vi "2D_scan.vi"(0 "X起始":dbl format="%#_13g", 1 "ERR X":errorcluster, 2 "模块路径":path=path "D:/Github/Motor_ctrl/3d_plot.py", 3 "ERR Y":errorcluster, 4 "Y起始":dbl format="%#_13g", 5 "X步长":dbl format="%#_13g", 6 "Y步长":dbl format="%#_13g", 9 "X终止":dbl format="%#_13g", 10 "Y终止":dbl format="%#_13g", 11 "COM X":refnum<visa-resource-name>, 12 "COM Keithley":refnum<visa-resource-name>, 14 "ERR Keithley":errorcluster, 15 "COM Y":refnum<visa-resource-name>) -> (13 "3D Plot lvclass Array out":refnum<class "3D Plot Datatype.lvclass">[](array[class]) caption="三维曲线lv类数组输出")   [LabVIEW 2018]
uses:
  <vilib>/Math Plots/3D Math Plots/3D Contour/3D Contour XCtrl/3D Contour.xctl
  <vilib>/Math Plots/3D Math Plots/3D Plot/3D Plot Datatype/3D Plot Datatype.lvclass
  <vilib>/Math Plots/3D Math Plots/3D Contour/3D Contour Datatype/Public/Plot Helper (Vector).vi
  <instrlib>/Keithley 648X Series/Keithley 648X Series.lvlib
  <vilib>/Math Plots/3D Math Plots/3D Contour/3D Contour Datatype/3D Contour Datatype.lvclass
panel:
  out "3D Contour":refnum<class "3D Plot Datatype.lvclass">[](xcontrol) caption="三维等高线"
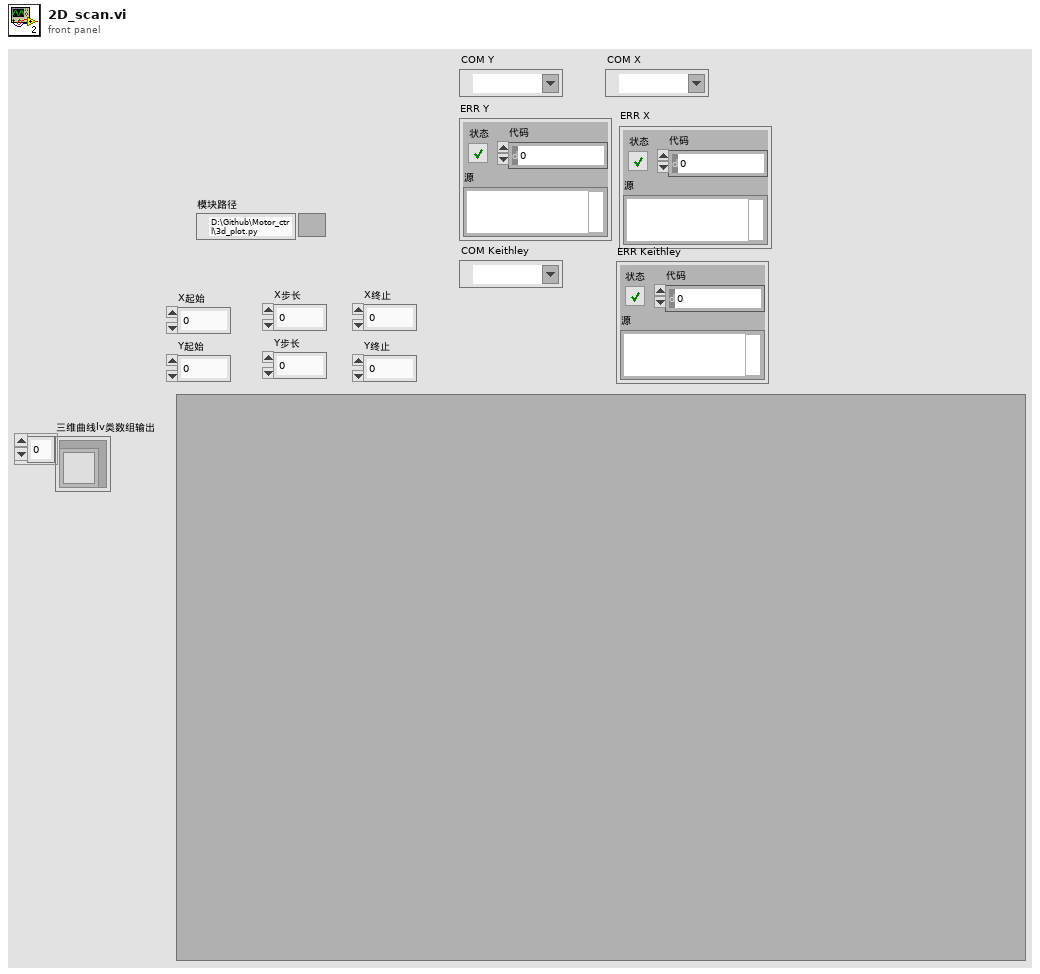
[diagram p1: front panel]
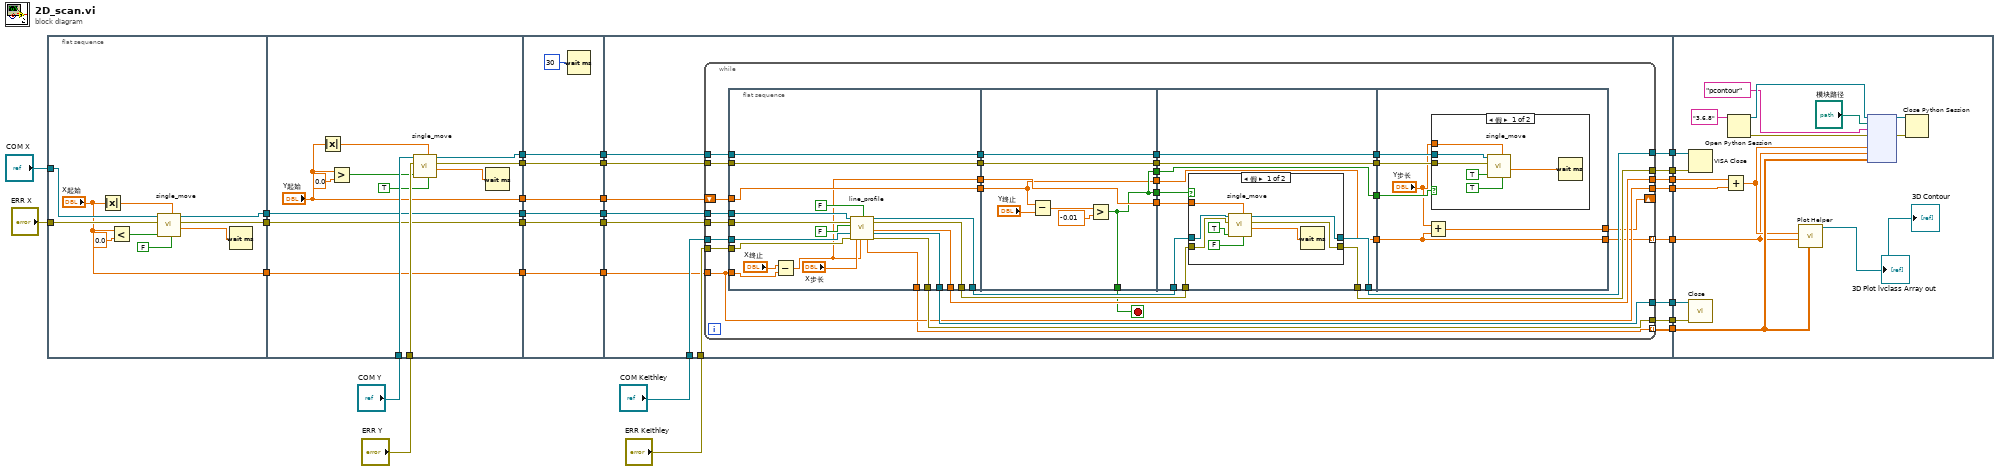
[diagram p0: block diagram]
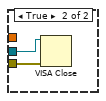
[diagram p3: hidden frame]
diagram:
  n1 = flat-sequence {
    tunnel: "COM X" -> [w39]
    tunnel: "ERR X" -> [w38]
    tunnel: [w37] -> w29
    tunnel: [w36] -> w28
    tunnel: ["X起始"] -> w27
    tunnel: "COM Y" -> [w52]
    tunnel: "ERR Y" -> [w51]
    tunnel: [w50] -> w26
    tunnel: [w49] -> w25
    tunnel: ["Y起始"] -> w24
    tunnel: [w48] -> w23
    tunnel: w29 -> [w48]
    tunnel: [w47] -> w22
    tunnel: w28 -> [w47]
    tunnel: [w42] -> w21
    tunnel: w27 -> [w42]
    tunnel: w26 -> [w59]
    tunnel: [w59] -> w20
    tunnel: w25 -> [w58]
    tunnel: [w58] -> w19
    tunnel: w24 -> [w57]
    tunnel: [w57] -> w18
    tunnel: w23 -> [w56]
    tunnel: [w56] -> w17
    tunnel: w22 -> [w55]
    tunnel: [w55] -> w16
    tunnel: w21 -> [w54]
    tunnel: [w54] -> w15
    tunnel: w20 -> [w75]
    tunnel: w19 -> [w74]
    tunnel: w18 -> [w73]
    tunnel: w17 -> [w72]
    tunnel: w16 -> [w71]
    tunnel: "COM Keithley" -> [w70]
    tunnel: "ERR Keithley" -> [w69]
    tunnel: [w68] -> w14
    tunnel: [w67] -> w13
    tunnel: [w66] -> w12
    tunnel: [w65] -> w11
    tunnel: [w64] -> w10
    tunnel: [w63] -> w9
    tunnel: w15 -> [w62]
    tunnel: [w61] -> w8
    tunnel: [w60] -> w7
    tunnel: w14 -> [w185]
    tunnel: w13 -> [w186]
    tunnel: w12 -> [w183]
    tunnel: w11 -> [w184]
    tunnel: w10 -> [w174]
    tunnel: w9 -> [w173]
    tunnel: w8 -> [w171]
    tunnel: w7 -> [w170]
    frame #0 {
      n2 = Absolute Value(x="X起始") -> (abs(x)=w32:dbl)
      n3 = Less?(x="X起始", y=0.0) -> (x < y?=w33:bool)
      n4 = call "single_move.vi"("COM In"=w39, "error In"=w38, "反向"=w33, "移动距离(mm)"=w32, "Y轴"=FALSE) -> ("VISA resource name out 2"=w37:refnum<visa-resource-name>, "error out 2"=w36:errorcluster, "总用时"=w30:dbl)  [unwired: 2 in]
      n5 = Wait (ms)(milliseconds to wait=w30) -> ()  [unwired: 1 out]
    }
    frame #1 {
      n6 = Absolute Value(x="Y起始") -> (abs(x)=w43:dbl)
      n7 = Greater?(x="Y起始", y=0.0) -> (0:w44:bool)
      n8 = call "single_move.vi"("COM In"=w52, "error In"=w51, "反向"=w44, "移动距离(mm)"=w43, "Y轴"=TRUE) -> ("VISA resource name out 2"=w50:refnum<visa-resource-name>, "error out 2"=w49:errorcluster, "总用时"=w40:dbl)  [unwired: 2 in]
      n9 = Wait (ms)(milliseconds to wait=w40) -> ()  [unwired: 1 out]
    }
    frame #2 {
      n10 = Wait (ms)(milliseconds to wait=u32 30 ("等待时间（毫秒）")) -> ()  [unwired: 1 out]
    }
    frame #3 {
      n11 = while {
        tunnel: w75 -> [w108]
        tunnel: w74 -> [w107]
        shift-right: [w78] -> _
        shift-left: w73 -> [w99]
        tunnel: w72 -> [w106]
        tunnel: w71 -> [w105]
        tunnel: w70 -> [w104]
        tunnel: w69 -> [w103]
        tunnel: [w95] -> w68
        tunnel: [w93] -> w67
        tunnel: [w102] -> w66
        tunnel: [w101] -> w65
        tunnel: [w97] -> w63 mode=indexing
        tunnel: [w100] -> w64
        tunnel: w62 -> [w98]
        tunnel: [w98] -> w61
        tunnel: [w77] -> w60 mode=indexing
        stop <- w84 stop-if-true
        n12 = flat-sequence {
          tunnel: w99 -> [w125]
          tunnel: w107 -> [w126]
          tunnel: w108 -> [w127]
          tunnel: [w127] -> w92
          tunnel: [w126] -> w90
          tunnel: [w125] -> w88
          tunnel: w106 -> [w124]
          tunnel: w105 -> [w123]
          tunnel: w104 -> [w122]
          tunnel: w103 -> [w121]
          tunnel: [w118] -> w96
          tunnel: [w117] -> w94
          tunnel: [w116] -> w102
          tunnel: [w115] -> w101
          tunnel: [w114] -> w97
          tunnel: [w113] -> w100
          tunnel: w98 -> [w111]
          tunnel: [w109] -> w87
          tunnel: w92 -> [w135]
          tunnel: [w135] -> w91
          tunnel: w90 -> [w134]
          tunnel: [w134] -> w89
          tunnel: w88 -> [w128]
          tunnel: w87 -> [w133]
          tunnel: [w133] -> w86
          tunnel: [w129] -> w85
          tunnel: [w129] -> w84
          tunnel: [w129] -> w79
          tunnel: [w128] -> w76
          tunnel: w91 -> [w145]
          tunnel: [w145] -> w83
          tunnel: w89 -> [w144]
          tunnel: [w144] -> w82
          tunnel: w96 -> [w143]
          tunnel: [w142] -> w95
          tunnel: w94 -> [w141]
          tunnel: [w140] -> w93
          tunnel: w86 -> [w139]
          tunnel: [w138] -> w81
          tunnel: w85 -> [w138]
          tunnel: [w137] -> w80
          tunnel: w79 -> [w136]
          tunnel: w76 -> [w137]
          tunnel: [w159] -> w78
          tunnel: w83 -> [w161]
          tunnel: w82 -> [w160]
          tunnel: w81 -> [w158]
          tunnel: w80 -> [w156]
          tunnel: [w156] -> w77
          frame #0 {
            n13 = Subtract(x="X终止", y=w111) -> (x-y=w109:dbl)
            n14 = call "line_profile.vi"("Motor COM in"=w124, "Motor error in"=w123, "Y轴"=FALSE, "Keithley COM In"=w122, "Keithley Error In"=w121, "步长"="X步长", "距离"=w109, "反向"=FALSE) -> ("电流数组"=w114:dbl[], "Motor COM out"=w118:refnum<visa-resource-name>, "Motor error out"=w117:errorcluster, "位移数组"=w113:dbl[], "Keithley COM out"=w116:refnum<visa-resource-name>, "Keithley Error out"=w115:errorcluster)  [unwired: 4 in, 2 out]
          }
          frame #1 {
            n15 = Subtract(x=w128, y="Y终止") -> (x-y=w131:dbl)
            n16 = Greater?(x=w131, y=-0.01) -> (0:w129:bool)
          }
          frame #2 {
            n17 = case shown="假" w136 {
              tunnel: w143 -> [w153 w154]
              tunnel: [w152 w154] -> w142
              tunnel: w141 -> [w151 w155]
              tunnel: [w150 w155] -> w140
              tunnel: w139 -> [w147 _]
              frame False {
                n18 = call "single_move.vi"("COM In"=w153, "error In"=w151, "反向"=TRUE, "移动距离(mm)"=w147, "Y轴"=FALSE) -> ("VISA resource name out 2"=w152:refnum<visa-resource-name>, "error out 2"=w150:errorcluster, "总用时"=w146:dbl)  [unwired: 2 in]
                n19 = Wait (ms)(milliseconds to wait=w146) -> ()  [unwired: 1 out]
              }
              frame True {
              }
            }
          }
          frame #3 {
            n20 = Add(x="Y步长", y=w156) -> (x+y=w159:dbl)
            n21 = case shown="假" w158 {
              tunnel: w161 -> [w167 w168]
              tunnel: w160 -> [w166 w169]
              tunnel: "Y步长" -> [w163 _]
              frame False {
                n22 = call "single_move.vi"("COM In"=w167, "error In"=w166, "反向"=TRUE, "移动距离(mm)"=w163, "Y轴"=TRUE) -> ("总用时"=w162:dbl)  [unwired: 2 in, 2 out]
                n23 = Wait (ms)(milliseconds to wait=w162) -> ()  [unwired: 1 out]
              }
              frame True {
                n24 = VISA Close(VISA resource name=w168, error in (no error)=w169) -> ()  [unwired: 1 out]
              }
            }
          }
        }
      }
    }
    frame #4 {
      n25 = VISA Close(VISA resource name=w185, error in (no error)=w186) -> ()  [unwired: 1 out]
      n26 = call <instrlib>:"Close.vi"("error in (no error)"=w184, "VISA resource name"=w183) -> ()  [unwired: 9 in, 1 out]
      n27 = Add(x=w174, y=w171) -> (x+y=w172:dbl[])
      n28 = Open Python Session(python version="3.6.8" ("Python版本")) -> (session out=w180:refnum<k35>, error out=w179:errorcluster)  [unwired: 2 in]
      n29 = call-poly <vilib>:"Plot Helper.vi"("z matrix"=w173, "y vector"=w170, "x vector"=w172) -> ("3D Plot lvclass Array out"=→"3D Contour" →"3D Plot lvclass Array out":refnum<class "3D Plot Datatype.lvclass">[])  [unwired: 3 in, 5 out]
      n30 = node(w180, "模块路径", "pcontour" ("函数名称"), w179, w172, w170, w173) -> (w178:refnum<k35>, w177:errorcluster)  [unwired: 5 in, 2 out]
      n31 = Close Python Session(session in=w178, error in=w177) -> ()  [unwired: 1 out]
    }
  }
